vi "FPGA_PPG_close.vi"(0 "resource_in":refnum<visa-resource-name>, 5 "error in (no error)":errorcluster) -> (19 "error out":errorcluster)   [LabVIEW 2014, in "NI-FPGA_PPG_Driver.lvlib"]
doc: "Close the connection to the FPGA target.\n\nContact: Falk Ziegler, eMail: ziegler@physik.uni-greifswald.de"
uses:
  NI-FPGA_PPG_Driver.lvlib
  FPGA_PPG_action_type.ctl
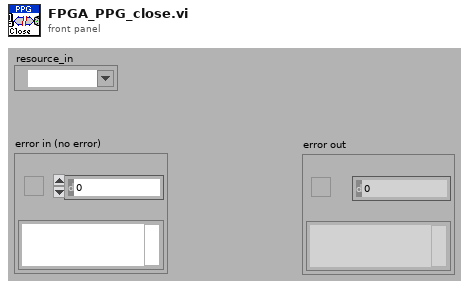
[diagram p1: front panel]
types:
  T1 = typedef "NI-FPGA_PPG_Driver.lvlib/FPGA_PPG_action_type.ctl" = enum16{"GET", "SET", "REMOVE"}
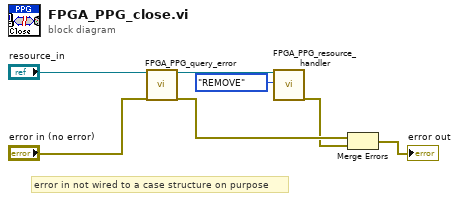
[diagram p0: block diagram]
diagram:
  # "error in not wired to a case structure on purpose"
  n1 = call "FPGA_PPG_query_error.vi"("resource_in"="resource_in", "error in (no error)"="error in (no error)") -> ("resource_out"=w7:refnum<visa-resource-name>, "error out"=w4:errorcluster)  [unwired: 16 in]
  n2 = call "FPGA_PPG_resource_handler.vi"("resource_in"=w7, "action"=FPGA_PPG_action_type."REMOVE") -> ("error out"=w2:errorcluster)  [unwired: 15 in, 2 out]
  n3 = Merge Errors(w4, w2) -> (→"error out":errorcluster)
